vi "Cover Rectangle Point to ROI.vi"(11 "Global Rectangle in":i32[](array[numeric])) -> (3 "ROI Array":i32[](array[numeric]))   [LabVIEW 2020]
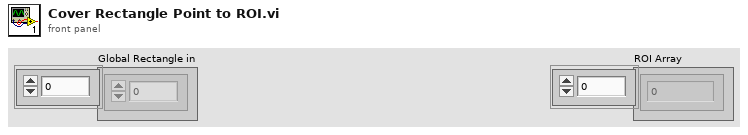
[diagram p1: front panel]
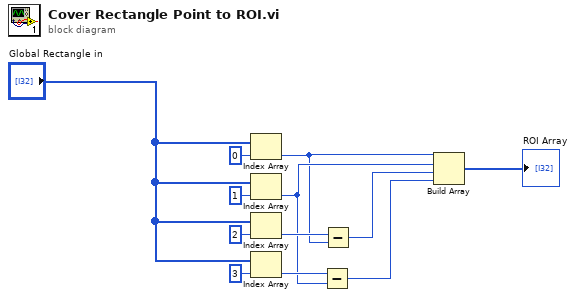
[diagram p0: block diagram]
diagram:
  n1 = Index Array(array="Global Rectangle in", index=0) -> (element=w4:i32)
  n2 = Index Array(array="Global Rectangle in", index=1) -> (element=w5:i32)
  n3 = Index Array(array="Global Rectangle in", index=2) -> (element=w7:i32)
  n4 = Index Array(array="Global Rectangle in", index=3) -> (element=w6:i32)
  n5 = Subtract(x=w6, y=w5) -> (x-y=w2:i32)
  n6 = Subtract(x=w7, y=w4) -> (x-y=w3:i32)
  n7 = Build Array(w4, w5, w3, w2) -> (→"ROI Array":i32[])
